vi "CheckMasterError.vi"(11 "String":string) -> ()   [LabVIEW 2012]
panel:
  out "T button?":bool
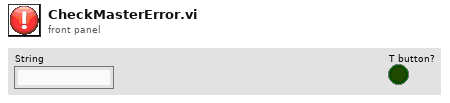
[diagram p1: front panel]
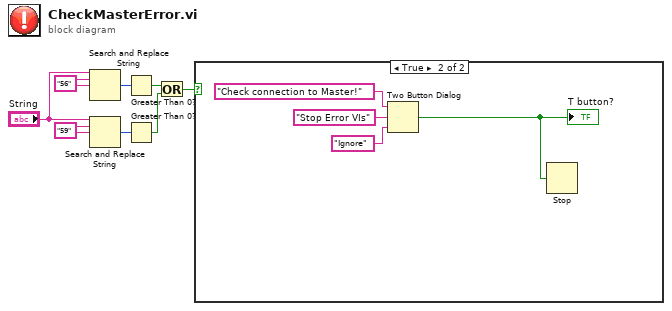
[diagram p0: block diagram]
diagram:
  w6 = "59" ("search string")
  w7 = "56" ("search string")
  n1 = Search and Replace String(input string="String", search string=w7, replace string=w7) -> (number of replacements=w5:i32)  [unwired: 5 in, 3 out]
  n2 = Search and Replace String(input string="String", search string=w6, replace string=w6) -> (number of replacements=w4:i32)  [unwired: 5 in, 3 out]
  n3 = Greater Than 0?(x=w5) -> (x > 0?=w2:bool)
  n4 = Greater Than 0?(x=w4) -> (x > 0?=w3:bool)
  n5 = Or(x=w2, y=w3) -> (x .or. y?=w1:bool)
  n6 = case shown="True" w1 {
    frame False {
    }
    frame True {
      n7 = Two Button Dialog(message="Check connection to Master!", 1:"Ignore" ("F button name (\"Cancel\")"), 2:"Stop Error VIs" ("T button name (\"OK\")")) -> (T button?=w9:bool)
      "T button?" <- w9
      n8 = Stop(stop? (T)=w9) -> ()
    }
  }
